vi "Release.vi"(8 "error in (no error)":errorcluster, 11 "LocalEventCollector in":refnum<class "LocalEventCollector.lvclass">) -> (0 "error out":errorcluster)   [LabVIEW 2020, in "Vecto.lvlib" / "LocalEventCollector.lvclass"]
uses:
  LocalEventCollector.lvclass
  LocalEventCollector.lvclass/LocalEventCollector.ctl
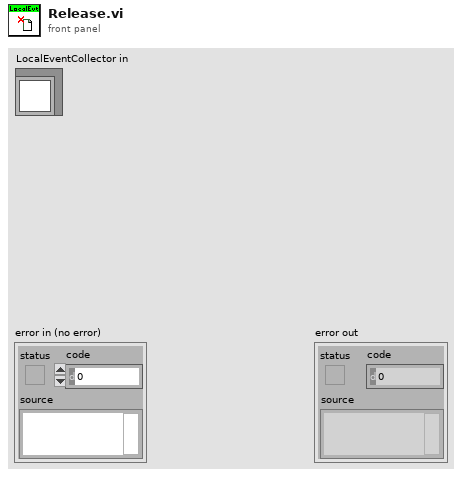
[diagram p1: front panel]
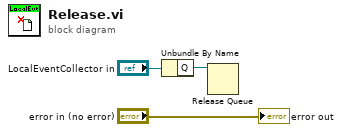
[diagram p0: block diagram]
diagram:
  n1 = Unbundle By Name("LocalEventCollector in") -> ("Q"=w1:refnum<queue>)
  n2 = Release Queue(queue=w1) -> ()  [unwired: 2 in, 3 out]
  "error out" <- "error in (no error)"
